vi "Combined10minPowerTrends.vi"() -> ()   [LabVIEW 2017, in "ImpedoDUO.lvlib"]
uses:
  ImpedoDUO.lvlib
panel:
  in  "Stop Button 2":bool
  in  "Stop Button":bool
  out "Waveform Chart Combined F403147 RealPower":sgl(graph)
  out "Waveform Chart F403147 RealPower ImpedoDUO":sgl(graph)
  out "Waveform Chart F403147 RealPower Vecto":sgl(graph)
  out "Waveform Chart Combined F403007 Voltage":sgl(graph)
  out "Waveform Chart F403007 Voltage ImpedoDUO":sgl(graph)
  out "Waveform Chart F403007 Voltage Vecto":sgl(graph)
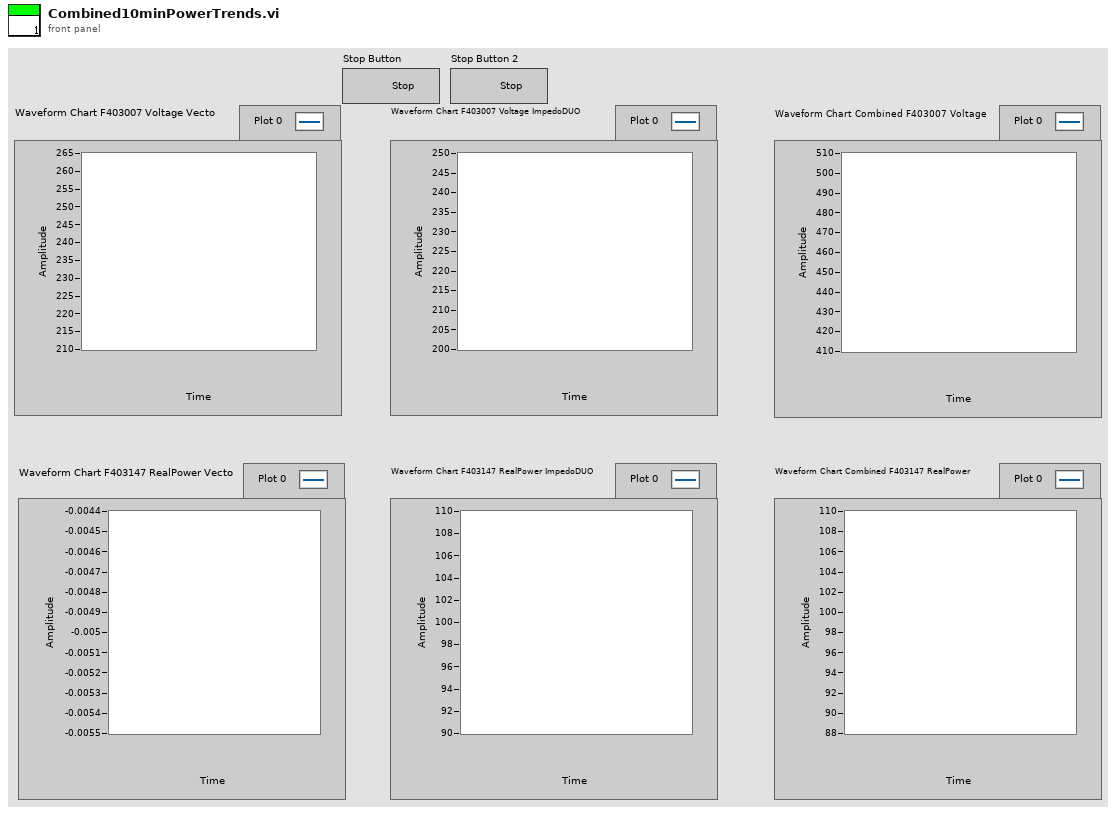
[diagram p1: front panel]
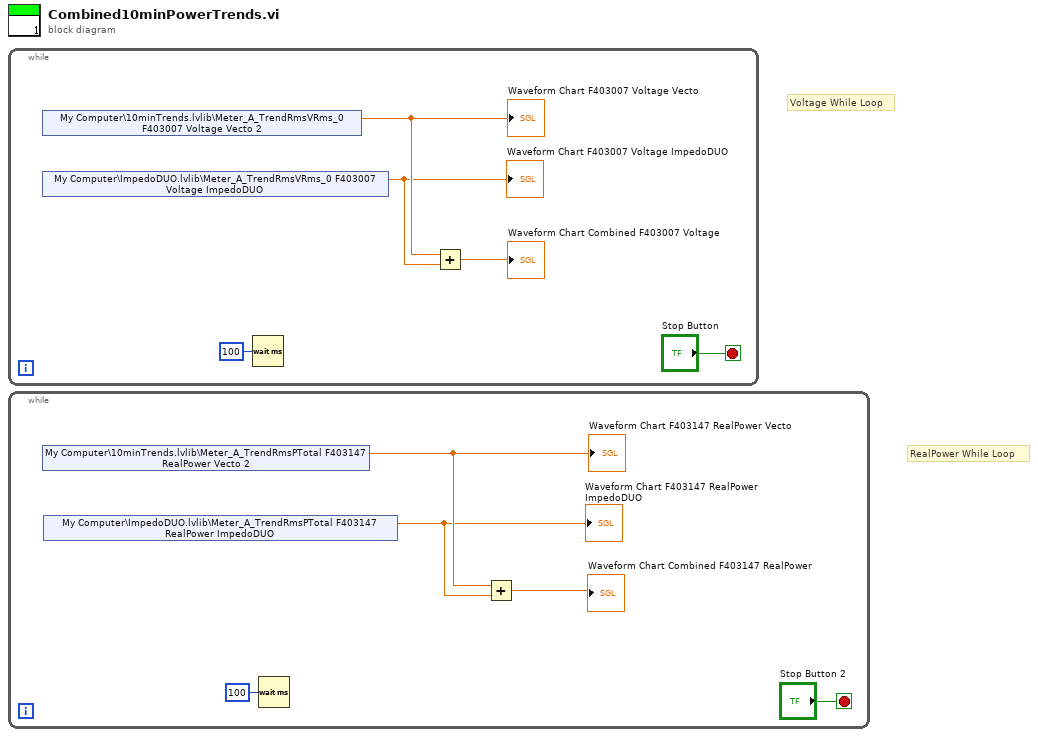
[diagram p0: block diagram]
diagram:
  # "RealPower While Loop"
  # "Voltage While Loop"
  n1 = while {
    stop <- "Stop Button" stop-if-true
    n2 = shared-variable "My Computer\\10minTrends.lvlib\\Meter_A_TrendRmsVRms_0 F403007 Voltage Vecto 2"() -> (w4:sgl)  [unwired: 1 in, 1 out]
    "Waveform Chart F403007 Voltage Vecto" <- w4
    n3 = shared-variable "My Computer\\ImpedoDUO.lvlib\\Meter_A_TrendRmsVRms_0 F403007 Voltage ImpedoDUO"() -> (w3:sgl)  [unwired: 1 in, 1 out]
    "Waveform Chart F403007 Voltage ImpedoDUO" <- w3
    n4 = Wait (ms)(milliseconds to wait=u32 100) -> ()  [unwired: 1 out]
    n5 = Add(x=w4, y=w3) -> (x+y=→"Waveform Chart Combined F403007 Voltage":sgl)
  }
  n6 = while {
    stop <- "Stop Button 2" stop-if-true
    n7 = shared-variable "My Computer\\10minTrends.lvlib\\Meter_A_TrendRmsPTotal F403147 RealPower Vecto 2"() -> (w9:sgl)  [unwired: 1 in, 1 out]
    "Waveform Chart F403147 RealPower Vecto" <- w9
    n8 = shared-variable "My Computer\\ImpedoDUO.lvlib\\Meter_A_TrendRmsPTotal F403147 RealPower ImpedoDUO"() -> (w8:sgl)  [unwired: 1 in, 1 out]
    "Waveform Chart F403147 RealPower ImpedoDUO" <- w8
    n9 = Wait (ms)(milliseconds to wait=u32 100) -> ()  [unwired: 1 out]
    n10 = Add(x=w9, y=w8) -> (x+y=→"Waveform Chart Combined F403147 RealPower":sgl)
  }
